vi "SetInvalidStatus.vi"(10 "valid":bool, 11 "props in":T1[](array[typedef])) -> (3 "props out":T1[](array[typedef]))   [LabVIEW 2017, in "EmsaDataEventCreator.lvlib"]
uses:
  <vilib>/addons/InsightCM/Devices/Shared/Emsa/EmsaDataEventCreator/EmsaDataEventCreator.lvlib
  <vilib>/addons/InsightCM/MessageBus/Base/controls/KeyValuePair.ctl
  <vilib>/addons/InsightCM/Utilities/PropertyHelpers/PropertyHelpers.lvlib
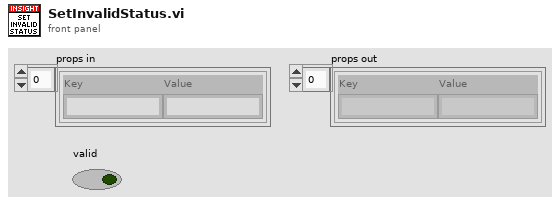
[diagram p1: front panel]
types:
  T1 = typedef "KeyValuePair.ctl" = cluster{"Key":string, "Value":string}
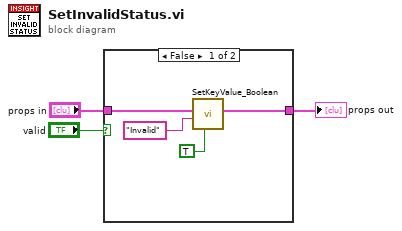
[diagram p0: block diagram]
diagram:
  n1 = case shown="False" "valid" {
    tunnel: [w6 w8] -> w2
    tunnel: "props in" -> [w7 w8]
    frame False {
      n2 = call <vilib>:"SetKeyValue_Boolean.vi"("value"=TRUE, "key"="Invalid", "key value pairs"=w7) -> ("key value pairs out"=w6:T1[])  [unwired: 8 in]
    }
    frame True {
    }
  }
  "props out" <- w2
